vi "I2C LCD Hello.vi"() -> ()   [LabVIEW 2020, in "CTI-Scratchpad.lvlib"]
uses:
  CTI-Scratchpad.lvlib
  CTI/I2C Number.ctl
  CTI/GPIO Number.ctl
  CTI-Peripheral/Grove I2C LCD/Grove I2C LCD.lvclass
  CTI/Session/Session.lvclass
  CTI/VisaComms/VisaComms.lvclass
  CTI/CTI.lvlib
panel:
  out "error out":errorcluster
  in  "Port":refnum<visa-resource-name>="COM4"
  in  "String":string="Hello LabVIEW!"
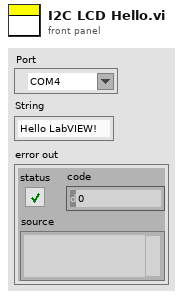
[diagram p1: front panel]
types:
  T1 = typedef "CTI.lvlib/GPIO Number.ctl" = i8
  T2 = typedef "CTI.lvlib/I2C Number.ctl" = i8
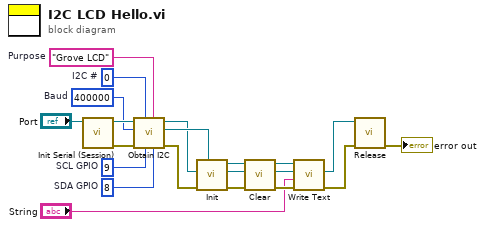
[diagram p0: block diagram]
diagram:
  w12 = T1 8  # SDA GPIO
  w13 = T1 9  # SCL GPIO
  w14 = "Grove LCD"  # Purpose
  w15 = T2 0  # I2C #
  w16 = u32 400000  # Baud
  n1 = call "Init Serial (Session).vi"("VISA resource name in"="Port") -> ("error out"=w17:errorcluster, "Session"=w18:refnum<class "Session.lvclass">)  [unwired: 9 in]
  n2 = call "Obtain I2C.vi"("SDA GPIO"=w12, "Purpose (\"I2C\")"=w14, "SCL GPIO"=w13, "I2C #"=w15, "error in (no error)"=w17, "Baud"=w16, "Session in"=w18) -> ("error out"=w9:errorcluster, "I2C"=w11:refnum<class "I2C.lvclass">, "Session out"=w10:refnum<class "Session.lvclass">)  [unwired: 2 in]
  n3 = call "Init.vi"("CTI.lvlib:I2C.lvclass"=w11, "error in (no error)"=w9, "Session In"=w10) -> ("error out"=w8:errorcluster, "Session Out"=w6:refnum<class "Session.lvclass">, "Grove I2C LCD out"=w7:refnum<class "Grove I2C LCD.lvclass">)  [unwired: 6 in]
  n4 = call-dynamic "Clear.vi"("error in (no error)"=w8, "Session In"=w6, "Character LCD in"=w7) -> ("error out"=w21:errorcluster, "Session Out"=w4:refnum<class "Session.lvclass">, "Character LCD out"=w5:refnum<class "Grove I2C LCD.lvclass">)  [unwired: 6 in]
  n5 = call-dynamic "Write Text.vi"("error in (no error)"=w21, "Text"="String", "Session In"=w4, "Character LCD in"=w5) -> ("error out"=w1:errorcluster, "Session Out"=w2:refnum<class "Session.lvclass">)  [unwired: 5 in, 1 out]
  n6 = call-dynamic "Release.vi"("error in (no error)"=w1, "Session in"=w2) -> ("error out"=→"error out":errorcluster)  [unwired: 9 in]
